vi "Baseline Monitor.vi"(0 "Baseline X":refnum<vi>, 1 "Baseline Y":refnum<vi>, 2 "Sweep Iter":refnum<vi>, 3 "Reference Triangle Wave":refnum<vi>, 4 "Input Triangle Wave":refnum<vi>, 5 "Modulator":refnum<vi>, 6 "Insta Mod":refnum<vi>, 7 "Normalized\nAdditive NMR\nY":refnum<vi>, 8 "Baseline\nSubtract":bool, 9 "Wings X":refnum<vi>, 10 "# of Sweeps":refnum<vi>, 11 "Wings Y":refnum<vi>, 13 "Wing Fit":refnum<vi>, 14 "Up/Down Ave X":refnum<vi>, 15 "Up/Down Ave Y":refnum<vi>) -> ()   [LabVIEW 2014]
panel:
  out "Background Subtracted / Wing Fit":cluster{"Y":dbl[], "Y":dbl[]}[](graph)
  out "# of Sweeps":i32
  out "Additive NMR":cluster{"Y":dbl[], "Y":dbl[]}[](graph)
  out "Instant NMR":cluster{"Y":dbl[], "Y":dbl[]}[](graph)
  out "Instant NMR":cluster{"Y":dbl[], "Y":dbl[]}[](graph)
  out "Sweep Iter":i32
  out "Sweep Averaging NMR":cluster{"Y":dbl[], "Y":dbl[]}[](graph)
  out "Modulator Sweeps":dbl[](graph)
  out "Input Triangle Wave":dynamicdata(graph)
  out "Last Baseline":cluster{"Y":dbl[], "Y":dbl[]}[](graph)
  # "VI Logic Pieces -- DO NOT TOUCH!!"
  # "If wings are not on edge, reset triangle wave rate"
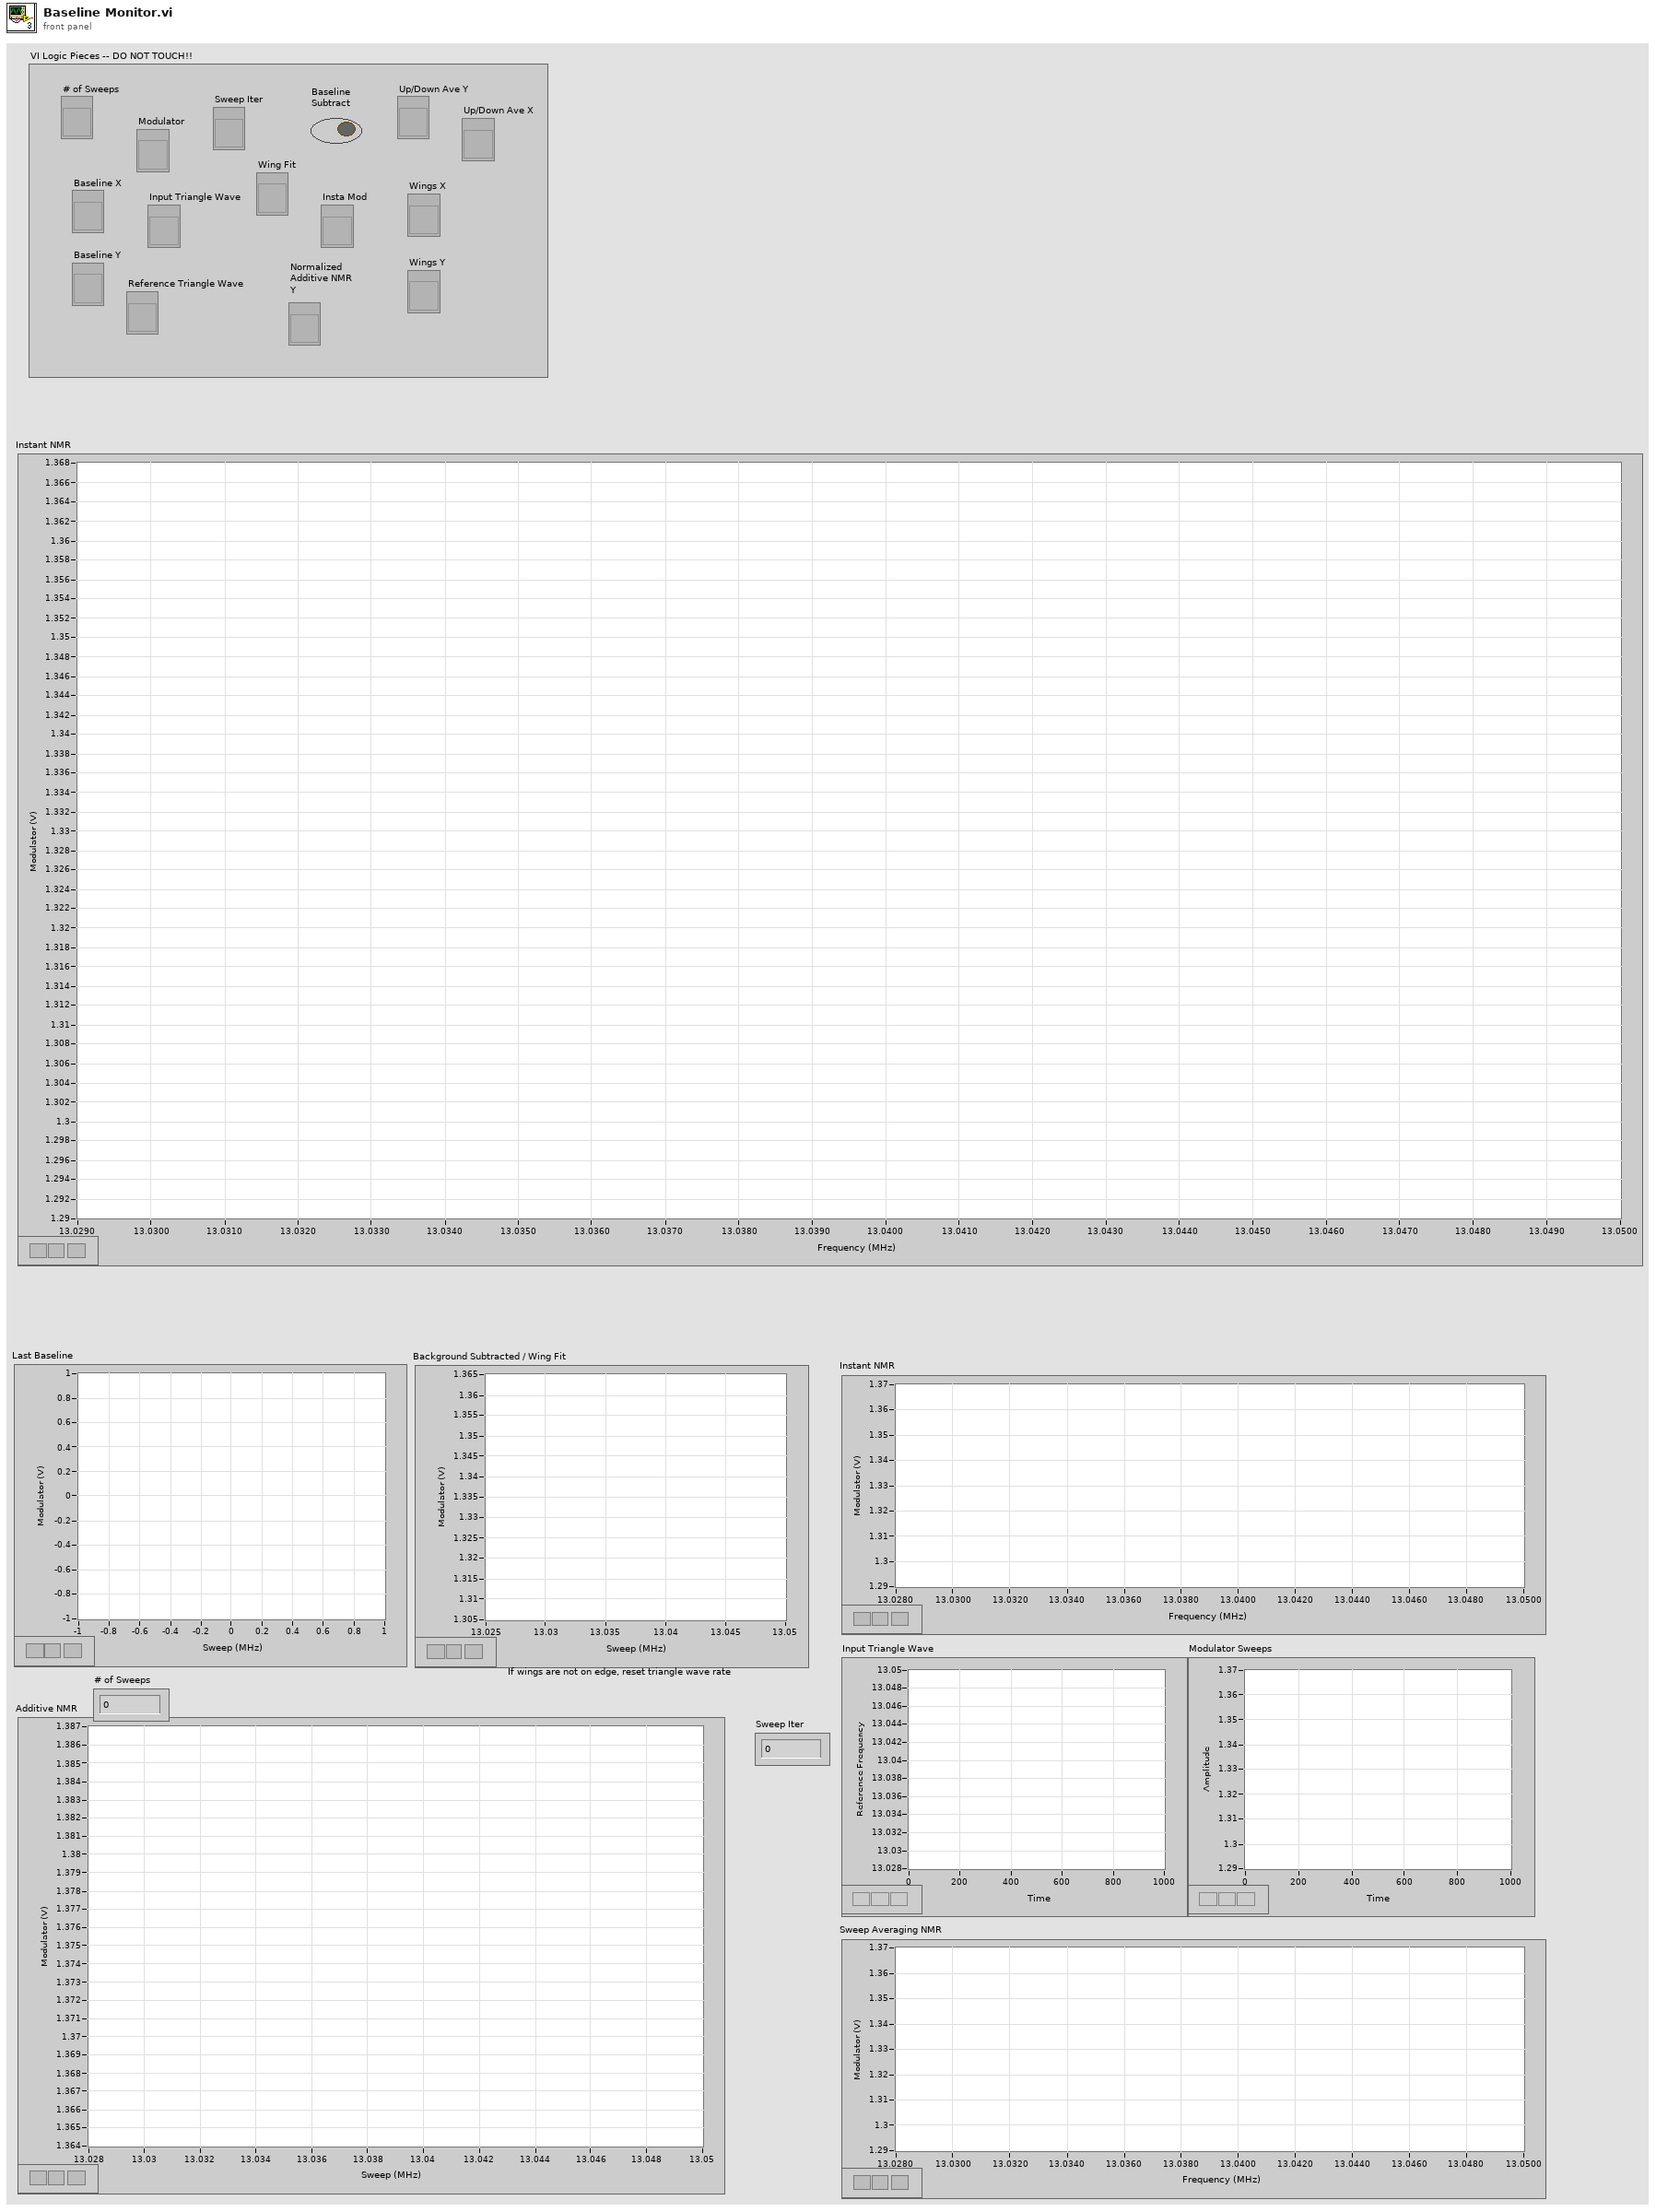
[diagram p1: front panel]
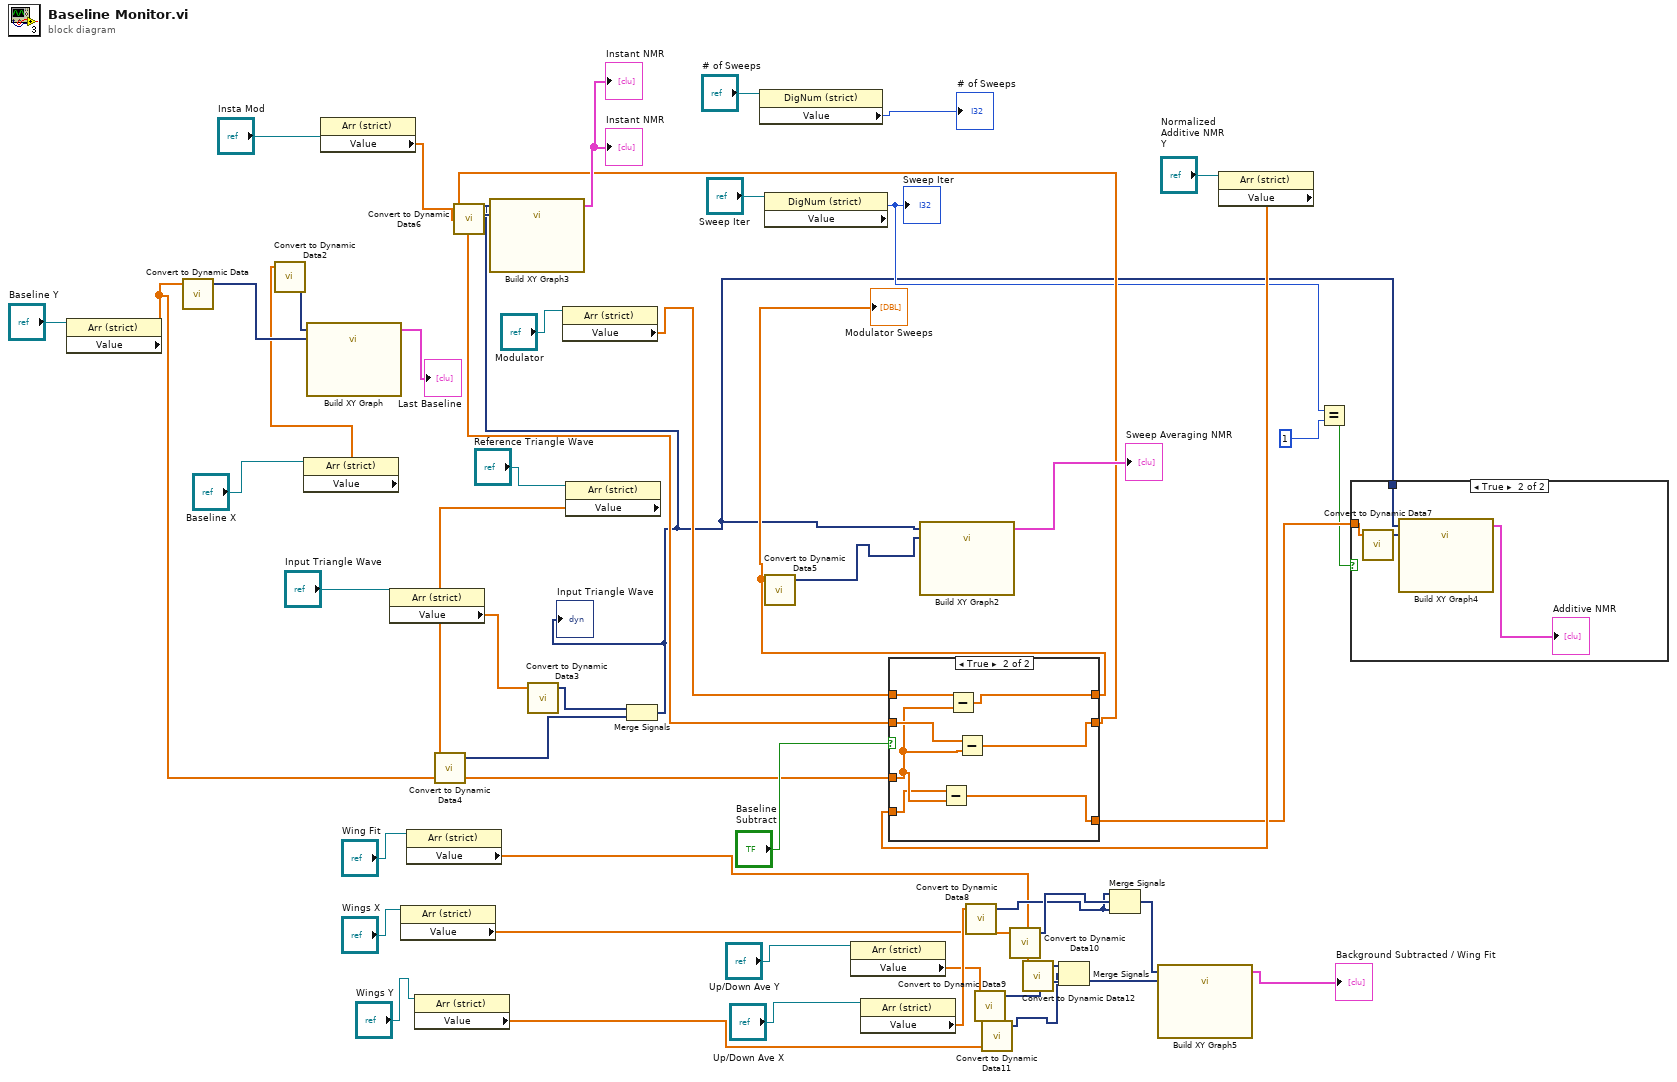
[diagram p0: block diagram]
diagram:
  n1 = property class="Arr (strict)"(reference="Baseline Y") -> ("Value"=w33:dbl[])  [unwired: 1 in, 2 out]
  n2 = call "Convert to Dynamic Data"("Array"=w33) -> ("Dynamic Data Type"=w52:dynamicdata)  [unwired: 3 in]
  n3 = property class="Arr (strict)"(reference="Baseline X") -> ("Value"=w46:dbl[])  [unwired: 1 in, 2 out]
  n4 = call "Convert to Dynamic Data2"("Array"=w46) -> ("Dynamic Data Type"=w47:dynamicdata)  [unwired: 3 in]
  n5 = call "Build XY Graph"("Y Input"=w52, "X Input"=w47) -> ("XY Graph"=→"Last Baseline":cluster{"Y":dbl[], "Y":dbl[]}[])  [unwired: 8 in, 1 out]
  n6 = property class="Arr (strict)"(reference="Insta Mod") -> ("Value"=w31:dbl[])  [unwired: 1 in, 2 out]
  n7 = property class="Arr (strict)"(reference="Input Triangle Wave") -> ("Value"=w42:dbl[])  [unwired: 1 in, 2 out]
  n8 = property class="Arr (strict)"(reference="Wings X") -> ("Value"=w8:dbl[])  [unwired: 1 in, 2 out]
  n9 = property class="Arr (strict)"(reference="Wing Fit") -> ("Value"=w2:dbl[])  [unwired: 1 in, 2 out]
  n10 = property class="Arr (strict)"(reference="Wings Y") -> ("Value"=w7:dbl[])  [unwired: 1 in, 2 out]
  n11 = call "Convert to Dynamic Data3"("Array"=w42) -> ("Dynamic Data Type"=w41:dynamicdata)  [unwired: 3 in]
  n12 = property class="Arr (strict)"(reference="Modulator") -> ("Value"=w32:dbl[])  [unwired: 1 in, 2 out]
  n13 = property class="Arr (strict)"(reference="Reference Triangle Wave") -> ("Value"=w40:dbl[])  [unwired: 1 in, 2 out]
  n14 = call "Convert to Dynamic Data4"("Array"=w40) -> ("Dynamic Data Type"=w39:dynamicdata)  [unwired: 3 in]
  n15 = Merge Signals(w41, w39) -> (w17:dynamicdata)
  "Input Triangle Wave" <- w17
  n16 = property class="DigNum (strict)"(reference="# of Sweeps") -> ("Value"=→"# of Sweeps":i32)  [unwired: 1 in, 2 out]
  n17 = property class="DigNum (strict)"(reference="Sweep Iter") -> ("Value"=w22:i32)  [unwired: 1 in, 2 out]
  "Sweep Iter" <- w22
  n18 = property class="Arr (strict)"(reference="Up/Down Ave Y") -> ("Value"=w9:dbl[])  [unwired: 1 in, 2 out]
  n19 = property class="Arr (strict)"(reference="Up/Down Ave X") -> ("Value"=w10:dbl[])  [unwired: 1 in, 2 out]
  n20 = call "Convert to Dynamic Data8"("Array"=w10) -> ("Dynamic Data Type"=w5:dynamicdata)  [unwired: 3 in]
  n21 = call "Convert to Dynamic Data9"("Array"=w9) -> ("Dynamic Data Type"=w4:dynamicdata)  [unwired: 3 in]
  n22 = call "Convert to Dynamic Data11"("Array"=w7) -> ("Dynamic Data Type"=w3:dynamicdata)  [unwired: 3 in]
  n23 = call "Convert to Dynamic Data10"("Array"=w8) -> ("Dynamic Data Type"=w6:dynamicdata)  [unwired: 3 in]
  n24 = call "Convert to Dynamic Data12"("Array"=w2) -> ("Dynamic Data Type"=w1:dynamicdata)  [unwired: 3 in]
  n25 = Merge Signals(w1, w3, w4) -> (w12:dynamicdata)
  n26 = Merge Signals(w5, w6, w5) -> (w13:dynamicdata)
  n27 = call "Build XY Graph5"("Y Input"=w12, "X Input"=w13) -> ("XY Graph"=→"Background Subtracted / Wing Fit":cluster{"Y":dbl[], "Y":dbl[]}[])  [unwired: 8 in, 1 out]
  n28 = property class="Arr (strict)"(reference="Normalized\nAdditive NMR\nY") -> ("Value"=w27:dbl[])  [unwired: 1 in, 2 out]
  n29 = case shown="True" "Baseline\nSubtract" {
    tunnel: w33 -> [_ w60]
    tunnel: w32 -> [w55 w62]
    tunnel: [w55 w58] -> w29
    tunnel: w31 -> [w54 w61]
    tunnel: [w54 w57] -> w30
    tunnel: w27 -> [w53 w59]
    tunnel: [w53 w56] -> w24
    frame False {
    }
    frame True {
      n30 = Subtract(x=w59, y=w60) -> (x-y=w56:dbl[])
      n31 = Subtract(x=w62, y=w60) -> (x-y=w58:dbl[])
      n32 = Subtract(x=w61, y=w60) -> (x-y=w57:dbl[])
    }
  }
  "Modulator Sweeps" <- w29
  n33 = call "Convert to Dynamic Data6"("Array"=w30) -> ("Dynamic Data Type"=w36:dynamicdata)  [unwired: 3 in]
  n34 = call "Build XY Graph3"("Y Input"=w36, "X Input"=w17) -> ("XY Graph"=→"Instant NMR" →"Instant NMR":cluster{"Y":dbl[], "Y":dbl[]}[])  [unwired: 8 in, 1 out]
  n35 = call "Convert to Dynamic Data5"("Array"=w29) -> ("Dynamic Data Type"=w16:dynamicdata)  [unwired: 3 in]
  n36 = call "Build XY Graph2"("Y Input"=w16, "X Input"=w17) -> ("XY Graph"=→"Sweep Averaging NMR":cluster{"Y":dbl[], "Y":dbl[]}[])  [unwired: 8 in, 1 out]
  n37 = Equal?(x=w22, y=1) -> (x = y?=w21:bool)
  n38 = case shown="True" w21 {
    tunnel: w24 -> [_ w64]
    tunnel: w17 -> [_ w63]
    frame False {
    }
    frame True {
      n39 = call "Convert to Dynamic Data7"("Array"=w64) -> ("Dynamic Data Type"=w66:dynamicdata)  [unwired: 3 in]
      n40 = call "Build XY Graph4"("Y Input"=w66, "X Input"=w63) -> ("XY Graph"=→"Additive NMR":cluster{"Y":dbl[], "Y":dbl[]}[])  [unwired: 8 in, 1 out]
    }
  }
